vi "set_sp_info.vi"(6 "yw":string, 8 "sp_shuoming":string, 9 "sp_yijian":string, 10 "id":string, 11 "lc_num":string) -> (0 "error 2":errorcluster caption="error", 3 "error":errorcluster)   [LabVIEW 2017, in "Lib_code.lvlib"]
uses:
  Lib_code.lvlib
panel:
  in  "error 4":errorcluster={"status"=TRUE, "code"=253, "source"="非法用户操作！"} caption="error"
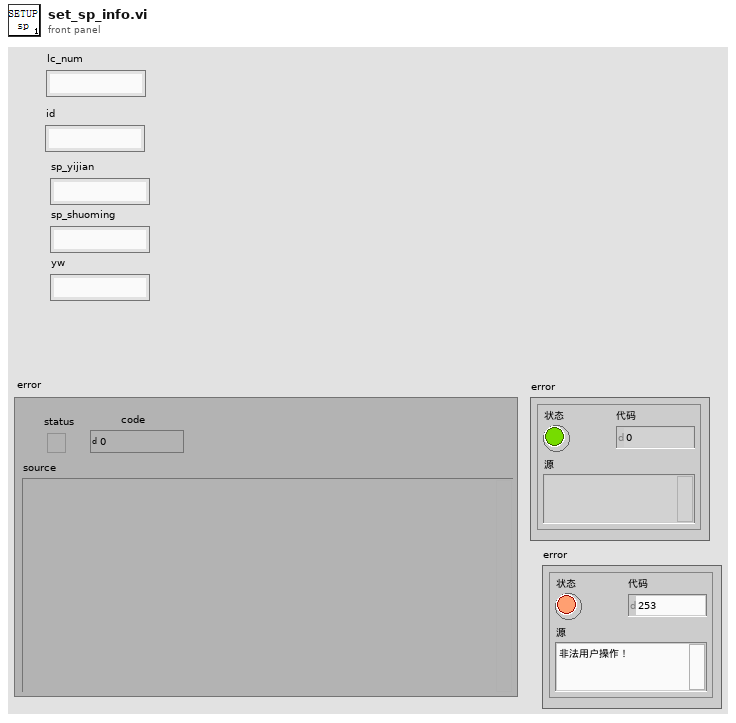
[diagram p1: front panel]
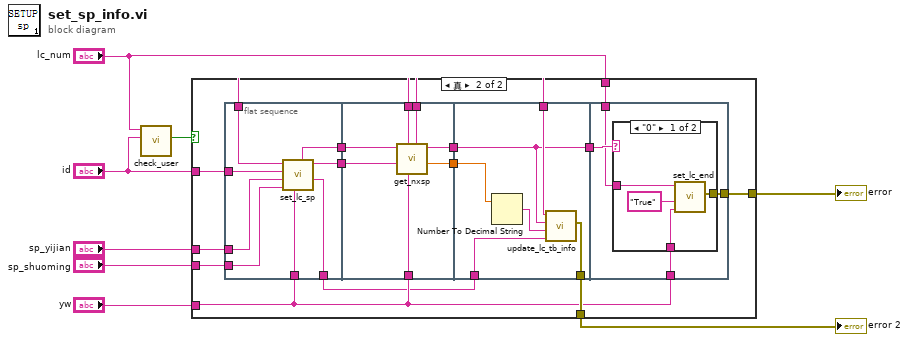
[diagram p0: block diagram]
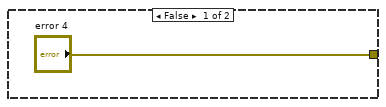
[diagram p2: hidden frame]
diagram:
  n1 = call "check_user.vi"("id"="id", "lc_num"="lc_num") -> ("check"=w1:bool)  [unwired: 8 in, 1 out]
  n2 = case shown="真" w1 {
    tunnel: "sp_yijian" -> [_ w17]
    tunnel: "sp_shuoming" -> [_ w16]
    tunnel: ["error 4" w15] -> w6
    tunnel: [_ w14] -> w5
    tunnel: "yw" -> [_ w13]
    tunnel: "lc_num" -> [_ w11]
    tunnel: "id" -> [_ w10]
    frame False {
    }
    frame True {
      n3 = flat-sequence {
        tunnel: [w30] -> w22
        tunnel: w11 -> [w29]
        tunnel: w10 -> [w28]
        tunnel: w17 -> [w27]
        tunnel: w16 -> [w26]
        tunnel: w13 -> [w25]
        tunnel: [w24] -> w21
        tunnel: [w23] -> w12
        tunnel: w22 -> [w32]
        tunnel: w13 -> [w36]
        tunnel: w21 -> [w37]
        tunnel: w11 -> [w35]
        tunnel: w10 -> [w34]
        tunnel: [w33] -> w20
        tunnel: [w31] -> w19
        tunnel: w11 -> [w43]
        tunnel: [w38] -> w18
        tunnel: [w42] -> w14
        tunnel: w12 -> [w41]
        tunnel: w20 -> [w39]
        tunnel: w19 -> [w38]
        tunnel: w18 -> [w47]
        tunnel: w11 -> [w46]
        tunnel: w13 -> [w45]
        tunnel: [w44] -> w15
        frame #0 {
          n4 = call "set_lc_sp.vi"("yw"=w25, "sp_shuoming"=w26, "sp_yijian"=w27, "id"=w28, "lc_num"=w29) -> ("cur_spnum"=w23:string, "cur_spsta"=w30:string, "fqren"=w24:string)  [unwired: 4 in]
        }
        frame #1 {
          n5 = call "get_nxsp.vi"("lc_num"=w35, "yw"=w36, "id"=w34, "Cur_state"=w32, "fqren"=w37) -> ("nx_state"=w33:dbl, "sp_gonghao"=w31:string)  [unwired: 4 in, 1 out]
        }
        frame #2 {
          n6 = Number To Decimal String(number=w39) -> (decimal integer string=w40:string)  [unwired: 1 in]
          n7 = call "update_lc_tb_info.vi"("cur_spnum"=w41, "nx_spsta"=w40, "nx_spren"=w38, "lc_num"=w43) -> ("error"=w42:errorcluster)  [unwired: 7 in]
        }
        frame #3 {
          n8 = case shown="\"0\"" w47 {
            tunnel: w46 -> [w49 _]
            tunnel: w45 -> [w48 _]
            tunnel: [w50 _] -> w44
            frame "0" {
              n9 = call "set_lc_end.vi"("yw"=w48, "state"="True", "lc_num"=w49) -> ("error"=w50:errorcluster)  [unwired: 8 in]
            }
            frame "真", Default {
            }
          }
        }
      }
    }
  }
  "error" <- w6
  "error 2" <- w5
